vi "Flow_Buffer_Dbl_VIG.vi"(7 "Operation":enum16{"get data", "set data", "initialize"}(ring)=enum."set data", 8 "error in":errorcluster, 9 "GPM":dbl[](array[numeric])=[0.0, 0.01403, 0.0282, 0.04999, 0.10258, 0.2127, 0.29025, 0.38705, 0.4802, 0.58116, 0.67343, 0.78891, 0.88241, 0.99458, 1.0892, 1.18752, 1.40024, 1.49696, 1.61641, 1.82395, 2.03827], 10 "Hz":dbl[](array[numeric])=[0.0, 3.61, 7.37, 13.09, 27.01, 55.78, 75.99, 100.94, 124.81, 150.52, 173.77, 202.7, 225.93, 253.45, 276.83, 301.27, 352.82, 375.82, 403.94, 453.6, 503.78], 11 "Freq":dbl) -> (0 "error out":errorcluster, 2 "Flow Hz":dbl, 3 "FlowGPH":dbl)   [LabVIEW 2018]
uses:
  <vilib>/Analysis/baseanly.llb/Mean (DBL).vi
  <vilib>/measure/macond.llb/FIR Filter for 1 Chan.vi
  <vilib>/gmath/NI_Gmath.lvlib
  <vilib>/measure/NI_MAPro.lvlib
  <vilib>/Analysis/NI_AALBase.lvlib
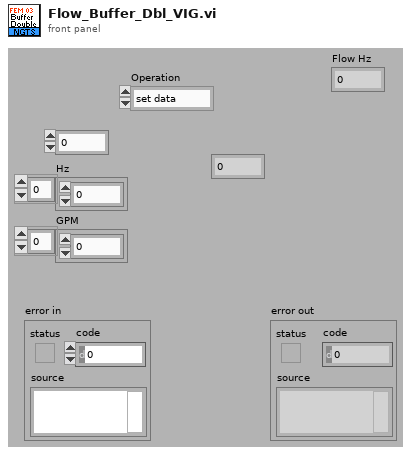
[diagram p1: front panel]
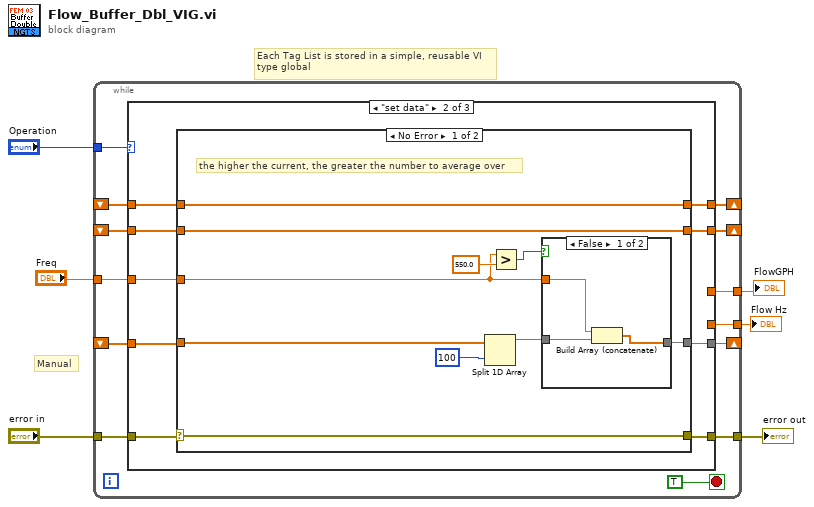
[diagram p0: block diagram]
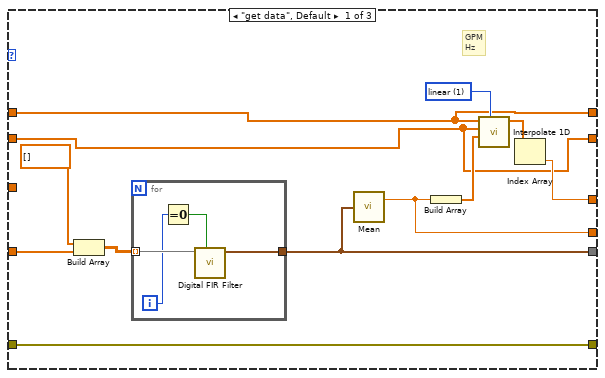
[diagram p2: hidden frame]
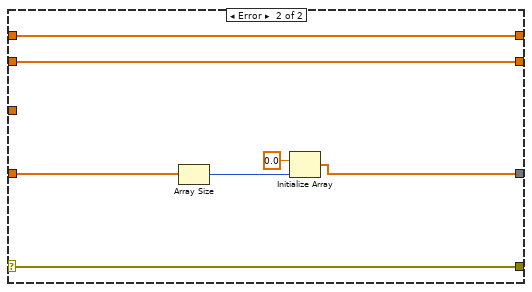
[diagram p4: hidden frame]
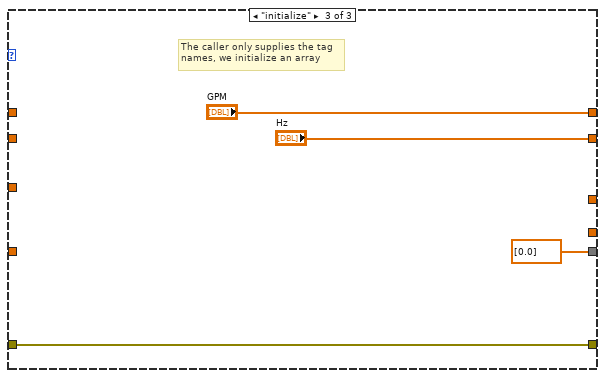
[diagram p5: hidden frame]
diagram:
  # "Manual"
  # "Each Tag List is stored in a simple, reusable VI\ntype global"
  n1 = while {
    tunnel: "Operation" -> [w19]
    tunnel: "Freq" -> [w17]
    tunnel: "error in" -> [w16]
    tunnel: [w15] -> w4
    shift-right: [w14] -> _
    shift-left: _ -> [w13]
    tunnel: [w12] -> w3
    shift-right: [w11] -> _
    shift-left: _ -> [w9]
    shift-right: [w10] -> _
    shift-left: _ -> [w8]
    tunnel: [w7] -> w1
    stop <- TRUE stop-if-true
    n2 = case shown="\"set data\"" w19 {
      tunnel: w17 -> [_ w42 _]
      tunnel: w16 -> [w31 w41 w69]
      tunnel: [w31 w40 w69] -> w15
      tunnel: [w23 w44 dbl[] [0.0] ("Array")] -> w14
      tunnel: w13 -> [w26 w43 _]
      tunnel: [w27 _ _] -> w12
      tunnel: [w22 w39 "GPM"] -> w11
      tunnel: [w21 w37 "Hz"] -> w10
      tunnel: w9 -> [w22 w38 _]
      tunnel: w8 -> [w21 w36 _]
      tunnel: [w20 _ _] -> w7
      frame "get data", Default {
        w30 = 1 items=["nearest", "linear", "spline", "cubic Hermite", "Lagrange"] ("method")
        # "GPM\nHz"
        n3 = Build Array(dbl[] [], w26) -> (w25:dbl[][])
        n4 = for {
          tunnel: w25 -> [w34] mode=indexing
          tunnel: [w35] -> w23
          i -> [w32]
          n5 = Equal To 0?(x=w32) -> (x = 0?=w33:bool)
          n6 = call-poly <vilib>:"Digital FIR Filter.vi"("reset filter"=w33, "signal in"=w34) -> ("signal out"=w35:waveform(dbl))  [unwired: 7 in, 2 out]
        }
        n7 = call-poly <vilib>:"Mean.vi"("X"=w23) -> ("mean"=w20:dbl)  [unwired: 1 out]
        n8 = Build Array(w20) -> (w28:dbl[])
        n9 = call <vilib>:"Interpolate 1D.vi"("method"=w30, "xi"=w28, "X"=w21, "Y"=w22) -> ("yi"=w29:dbl[])  [unwired: 5 in, 2 out]
        n10 = Index Array(array=w29) -> (element=w27:dbl)  [unwired: 1 in]
      }
      frame "set data" {
        n11 = case shown="No Error" w41 {
          selector: w41 -> [w51 w65]
          tunnel: [w54 w61] -> w44
          tunnel: w43 -> [w53 w64]
          tunnel: w42 -> [w47 _]
          tunnel: [w51 w65] -> w40
          tunnel: [w50 w60] -> w39
          tunnel: w38 -> [w50 w60]
          tunnel: [w49 w59] -> w37
          tunnel: w36 -> [w49 w59]
          frame No Error {
            # "the higher the current, the greater the number to average over"
            n12 = Split 1D Array(array=w53, index=100) -> (first subarray=w52:dbl[])  [unwired: 1 out]
            n13 = Greater?(x=w47, y=550.0) -> (0:w46:bool)
            n14 = case shown="False" w46 {
              tunnel: [w57 w58] -> w54
              tunnel: w52 -> [w56 w58]
              tunnel: w47 -> [w55 _]
              frame False {
                n15 = Build Array (concatenate)(w55, w56) -> (w57:dbl[])
              }
              frame True {
              }
            }
          }
          frame Error {
            n16 = Array Size(array=w64) -> (size(s)=w63:i32)
            n17 = Initialize Array(0.0 ("element"), w63) -> (w61:dbl[])
          }
        }
      }
      frame "initialize" {
        # "The caller only supplies the tag\nnames, we initialize an array"
      }
    }
  }
  "error out" <- w4
  "FlowGPH" <- w3
  "Flow Hz" <- w1
